vi "cw_2_8.vi"() -> ()   [LabVIEW 2022 SP3]
uses:
  <vilib>/numeric/Random Number (Range) DBL.vi
panel:
  out "concatenated string":string
  in  "stop":bool
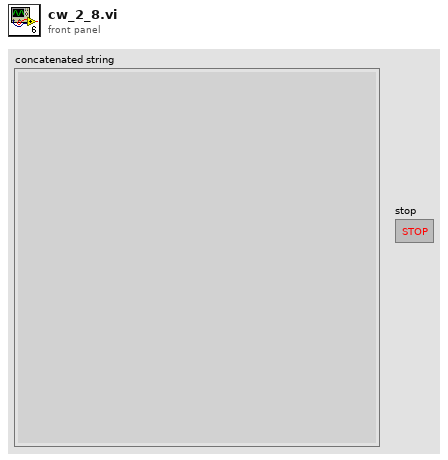
[diagram p1: front panel]
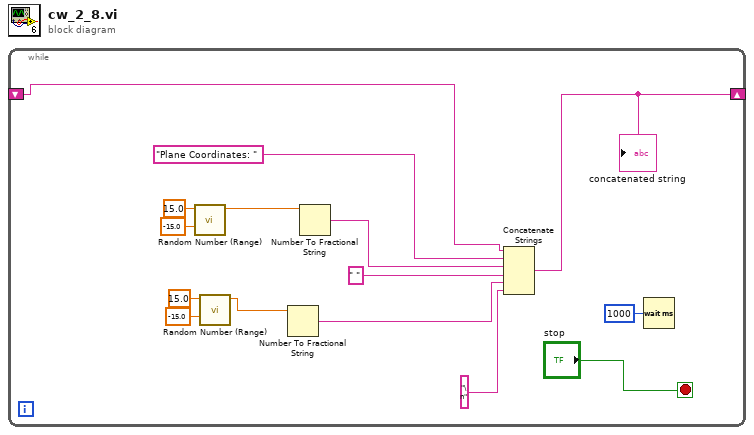
[diagram p0: block diagram]
diagram:
  n1 = while {
    shift-right: [w7] -> _
    shift-left: _ -> [w6]
    stop <- "stop" stop-if-true
    n2 = call-poly <vilib>:"Random Number (Range).vi"("lower bound (0)"=-15.0, "upper bound (100)"=15.0) -> ("number"=w10:dbl)  [unwired: 9 in]
    n3 = call-poly <vilib>:"Random Number (Range).vi"("lower bound (0)"=-15.0, "upper bound (100)"=15.0) -> ("number"=w9:dbl)  [unwired: 9 in]
    n4 = Number To Fractional String(number=w9) -> (F-format string=w4:string)  [unwired: 3 in]
    n5 = Number To Fractional String(number=w10) -> (F-format string=w2:string)  [unwired: 3 in]
    n6 = Concatenate Strings(w6, "Plane Coordinates: " ("string"), w2, " " ("string"), w4, "\n" ("string")) -> (w7:string)
    "concatenated string" <- w7
    n7 = Wait (ms)(milliseconds to wait=u32 1000) -> ()  [unwired: 1 out]
  }
